vi "CDMA_RxFilter.vi"(8 "error in (no error)":errorcluster caption="错误输入（无错误）", 9 "sampleRate":dbl, 10 "rx_data":cdb[](array[numeric]), 11 "Path":path) -> (0 "error out":errorcluster caption="错误输出", 2 "rxData":cdb[](array[numeric]), 3 "Path Out":path)   [LabVIEW 2015]
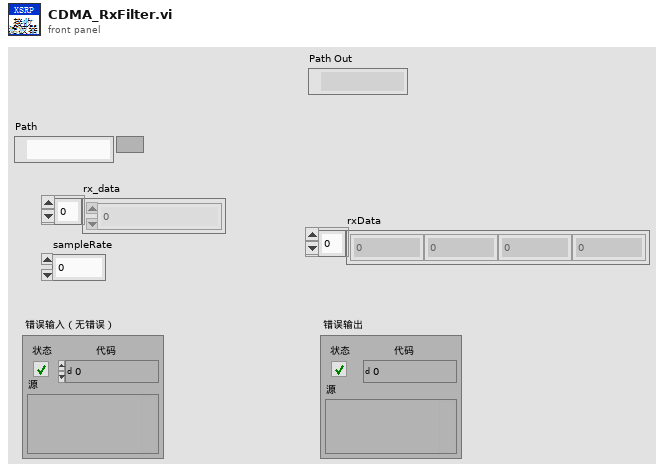
[diagram p1: front panel]
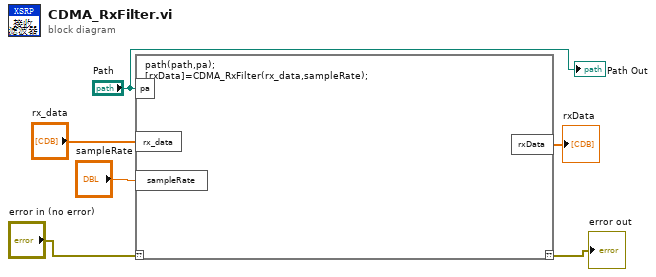
[diagram p0: block diagram]
diagram:
  n1 = script code="path(path,pa);\n[rxData]=CDMA_RxFilter(rx_data,sampleRate);"("??"="error in (no error)", "pa"="Path", "rx_data"="rx_data", "sampleRate"="sampleRate") -> ("??"=→"error out":errorcluster, "rxData"=→"rxData":cdb[])
  "Path Out" <- "Path"
